vi "JonHelpMay.vi"() -> ()   [LabVIEW 2015]
uses:
  <vilib>/Instr/_visa.llb/VISA Configure Serial Port (Instr).vi
  <vilib>/Utility/file.llb/Read Delimited Spreadsheet (DBL).vi
  <vilib>/Utility/file.llb/Read Delimited Spreadsheet (I64).vi
  <vilib>/Utility/file.llb/Write Delimited Spreadsheet (I64).vi
  <vilib>/Utility/file.llb/Write Delimited Spreadsheet (DBL).vi
panel:
  out "Waveform Graph":cluster{"first row":dbl[]}[](graph)
  out "Array 2":u8[](array[numeric])
  out "Array":u8[](array[numeric])
  in  "Stop Button":bool
  in  "VISA resource name":refnum<visa-resource-name>
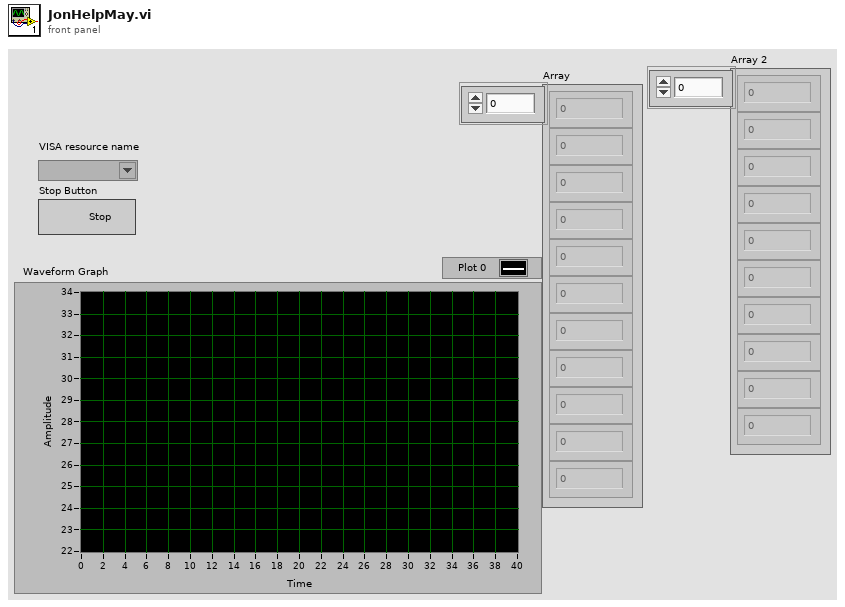
[diagram p1: front panel]
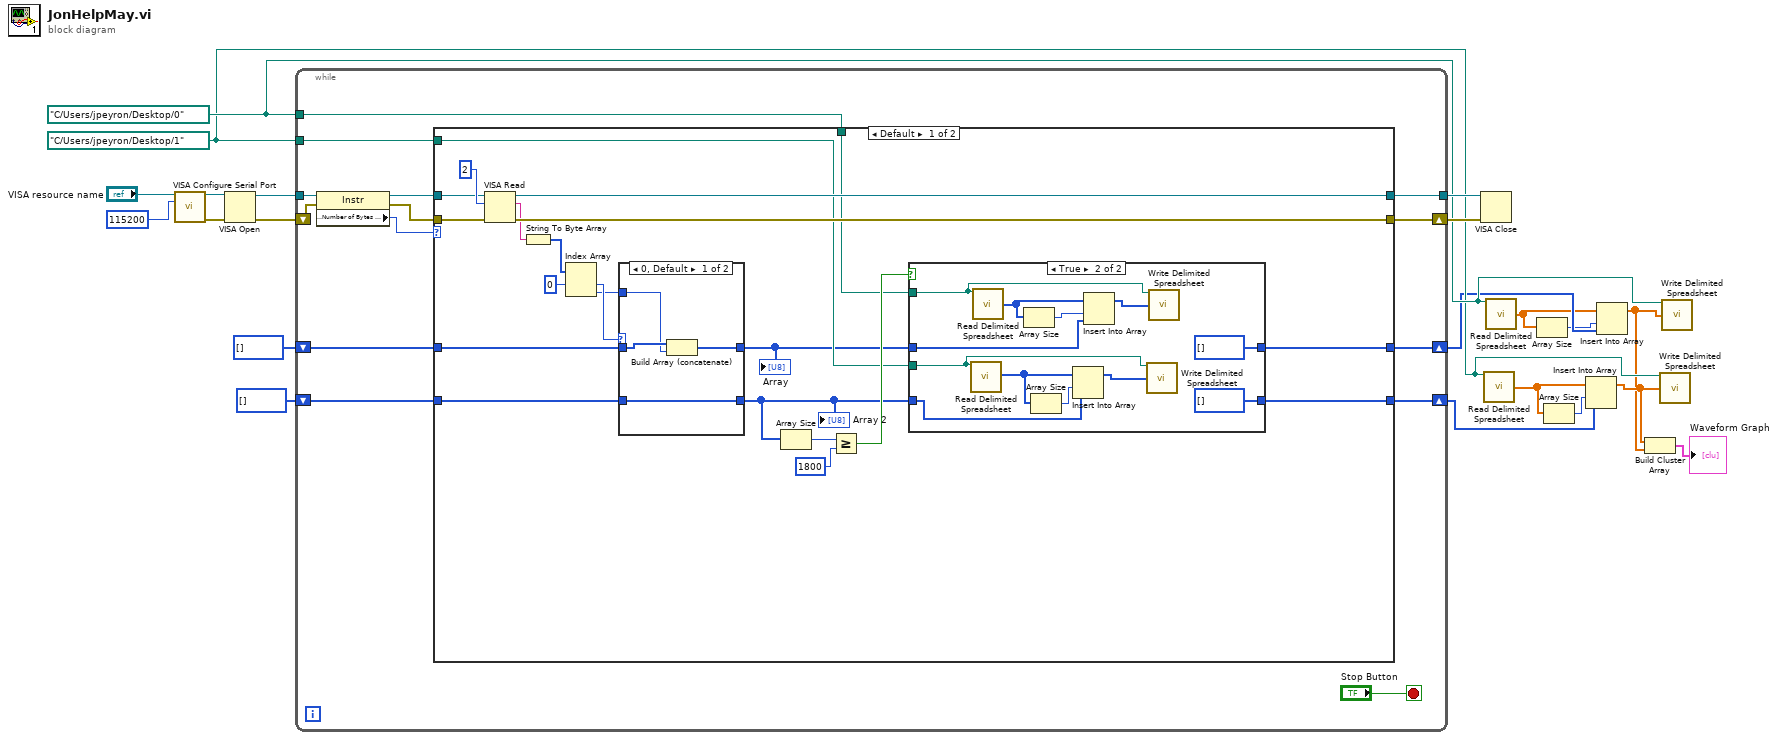
[diagram p0: block diagram]
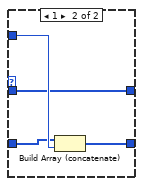
[diagram p3: hidden frame]
diagram:
  w10 = path "C:/Users/jpeyron/Desktop/1" ("file path (dialog if empty)")
  w11 = path "C:/Users/jpeyron/Desktop/0" ("file path (dialog if empty)")
  n1 = call-poly "VISA Configure Serial Port"("VISA resource name"="VISA resource name", "baud rate (9600)"=u32 115200) -> ("VISA resource name out"=w21:refnum<visa-resource-name>, "error out"=w20:errorcluster)  [unwired: 12 in]
  n2 = VISA Open(error in (no error)=w20, VISA resource name=w21) -> (VISA resource name=w17:refnum<visa-resource-name>, error out=w16:errorcluster)  [unwired: 3 in]
  n3 = while {
    tunnel: w17 -> [w34]
    shift-right: [w31] -> w15
    shift-left: w16 -> [w33]
    tunnel: [w28] -> w14
    shift-right: [w27] -> w8
    shift-left: u8[] [] -> [w26]
    shift-right: [w24] -> w7
    shift-left: u8[] [] -> [w25]
    tunnel: w11 -> [w23]
    tunnel: w10 -> [w22]
    stop <- "Stop Button" stop-if-true
    n4 = property class="Instr"(reference=w34, error in=w33) -> (reference out=w29:refnum<visa-resource-name>, error out=w32:errorcluster, "Serial Settings:Number of Bytes at Serial Port"=w30:u32)
    n5 = case shown="Default" w30 {
      tunnel: w32 -> [w56 w81]
      tunnel: [w55 w81] -> w31
      tunnel: w29 -> [w53 w82]
      tunnel: [w52 w82] -> w28
      tunnel: [w36 w80] -> w27
      tunnel: w26 -> [w45 w80]
      tunnel: w25 -> [w47 w79]
      tunnel: [w37 w79] -> w24
      tunnel: w23 -> [w41 _]
      tunnel: w22 -> [w40 _]
      frame Default {
        n6 = VISA Read(VISA resource name=w53, byte count=u32 2, error in (no error)=w56) -> (VISA resource name out=w52:refnum<visa-resource-name>, read buffer=w51:string, error out=w55:errorcluster)  [unwired: 1 out]
        n7 = String To Byte Array(string=w51) -> (unsigned byte array=w49:u8[])
        n8 = Index Array(array=w49, index #1=0 ("index")) -> (element #1=w48:u8, element #2=w46:u8)  [unwired: 1 in]
        n9 = case shown="0, Default" w48 {
          tunnel: w47 -> [w74 w75]
          tunnel: w46 -> [w73 w78]
          tunnel: [w71 w77] -> w38
          tunnel: [w72 w75] -> w39
          tunnel: w45 -> [w71 w76]
          frame 0, Default {
            n10 = Build Array (concatenate)(w74, w73) -> (w72:u8[])
          }
          frame 1 {
            n11 = Build Array (concatenate)(w76, w78) -> (w77:u8[])
          }
        }
        "Array" <- w39
        "Array 2" <- w38
        n12 = Array Size(array=w38) -> (size(s)=w44:i32)
        n13 = Greater Or Equal?(x=w44, y=1800) -> (x >= y?=w42:bool)
        n14 = case shown="True" w42 {
          tunnel: w41 -> [_ w66]
          tunnel: w40 -> [_ w65]
          tunnel: w39 -> [w58 w68]
          tunnel: w38 -> [w57 w63]
          tunnel: [w58 u8[] []] -> w37
          tunnel: [w57 u8[] []] -> w36
          frame False {
          }
          frame True {
            n15 = call-poly <vilib>:"Read Delimited Spreadsheet.vi"("file path (dialog if empty)"=w65) -> ("first row"=w61:i64[])  [unwired: 9 in, 5 out]
            n16 = call-poly <vilib>:"Read Delimited Spreadsheet.vi"("file path (dialog if empty)"=w66) -> ("first row"=w70:i64[])  [unwired: 9 in, 5 out]
            n17 = Array Size(array=w70) -> (size(s)=w69:i32)
            n18 = Array Size(array=w61) -> (size(s)=w64:i32)
            n19 = Insert Into Array(array=w61, index=w64, new element=w63) -> (w62:i64[])
            n20 = Insert Into Array(array=w70, index=w69, new element=w68) -> (w67:i64[])
            n21 = call-poly <vilib>:"Write Delimited Spreadsheet.vi"("file path (dialog if empty)"=w65, "1D data"=w62) -> ()  [unwired: 12 in, 2 out]
            n22 = call-poly <vilib>:"Write Delimited Spreadsheet.vi"("file path (dialog if empty)"=w66, "1D data"=w67) -> ()  [unwired: 12 in, 2 out]
          }
        }
      }
      frame 0 {
      }
    }
  }
  n23 = VISA Close(VISA resource name=w14, error in (no error)=w15) -> ()  [unwired: 1 out]
  n24 = call-poly <vilib>:"Read Delimited Spreadsheet.vi"("file path (dialog if empty)"=w10) -> ("first row"=w4:dbl[])  [unwired: 9 in, 5 out]
  n25 = call-poly <vilib>:"Read Delimited Spreadsheet.vi"("file path (dialog if empty)"=w11) -> ("first row"=w5:dbl[])  [unwired: 9 in, 5 out]
  n26 = Array Size(array=w5) -> (size(s)=w6:i32)
  n27 = Array Size(array=w4) -> (size(s)=w9:i32)
  n28 = Insert Into Array(array=w4, index=w9, new element=w8) -> (w3:dbl[])
  n29 = Insert Into Array(array=w5, index=w6, new element=w7) -> (w2:dbl[])
  n30 = Build Cluster Array(w3, w2) -> (→"Waveform Graph":cluster{"first row":dbl[]}[])
  n31 = call-poly <vilib>:"Write Delimited Spreadsheet.vi"("file path (dialog if empty)"=w10, "1D data"=w3) -> ()  [unwired: 12 in, 2 out]
  n32 = call-poly <vilib>:"Write Delimited Spreadsheet.vi"("file path (dialog if empty)"=w11, "1D data"=w2) -> ()  [unwired: 12 in, 2 out]
